vi "Write FunctionError.vi"(8 "error in (no error)":errorcluster, 10 "FunctionError":string, 11 "LoggingWrapper in":refnum<class "LoggingWrapper.lvclass">) -> (0 "error out":errorcluster, 3 "LoggingWrapper out":refnum<class "LoggingWrapper.lvclass">)   [LabVIEW 2022 SP3, in "Logger.lvlib" / "LoggingWrapper.lvclass"]
uses:
  LoggingWrapper.lvclass
  LoggingWrapper.lvclass/LoggingWrapper.ctl
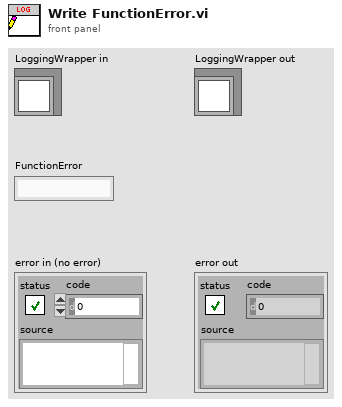
[diagram p1: front panel]
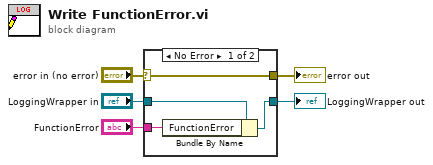
[diagram p0: block diagram]
diagram:
  n1 = case shown="No Error" "error in (no error)" {
    selector: "error in (no error)" -> [w9 w10]
    tunnel: [w9 w10] -> w4
    tunnel: [w7 w11] -> w2
    tunnel: "LoggingWrapper in" -> [w8 w11]
    tunnel: "FunctionError" -> [w6 _]
    frame No Error {
      n2 = Bundle By Name(cluster=w8, "FunctionError"=w6) -> (w7:refnum<class "LoggingWrapper.lvclass">)
    }
    frame Error {
    }
  }
  "error out" <- w4
  "LoggingWrapper out" <- w2
